vi "Send Set Power Setpoints.vi"(7 "Message Priority (Normal)":T1=enum."Normal", 8 "error in (no error)":errorcluster, 9 "Right Power Setpoint":dbl(slide) min=-1.0 max=1.0 step=0.1 scale=-1.0..1.0, 10 "Left Power Setpoint":dbl(slide) min=-1.0 max=1.0 step=0.1 scale=-1.0..1.0, 11 "Message Enqueuer":refnum<class "Message Enqueuer.lvclass">) -> (0 "error out":errorcluster, 3 "Message Enqueuer out":refnum<class "Message Enqueuer.lvclass">)   [LabVIEW 2014, in "Logical Systems.lvlib" / "Drive Train.lvlib" / "Set Power Setpoints Msg.lvclass"]
doc: "This VI sends the message to an actor."
uses:
  Set Power Setpoints Msg.lvclass
  <vilib>/ActorFramework/Message Enqueuer/Message Enqueuer.lvclass
  <vilib>/ActorFramework/Message Enqueuer/Message Priority.ctl
  Set Power Setpoints Msg.lvclass/Set Power Setpoints Msg.ctl
  <vilib>/ActorFramework/Message Enqueuer/Message Enqueuer.lvclass/Message Enqueuer.ctl
  <vilib>/ActorFramework/Message Priority Queue/Priority Enqueue.vi
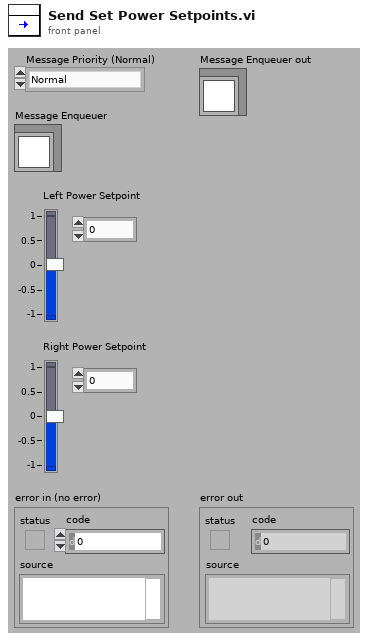
[diagram p1: front panel]
types:
  T1 = typedef "Actor Framework.lvlib/Message Enqueuer.lvclass/Message Priority.ctl" = enum16{"Low", "Normal", "High"}
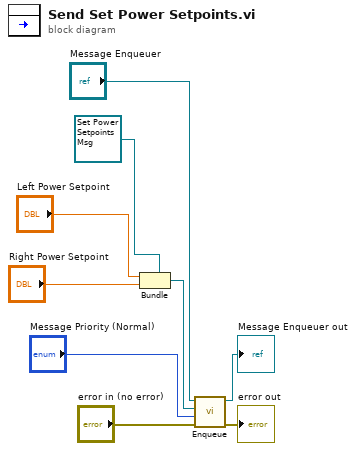
[diagram p0: block diagram]
diagram:
  n1 = Bundle(cluster=refnum<class "Set Power Setpoints Msg.lvclass"> refnum ("Object"), "Left Power Setpoint", "Right Power Setpoint") -> (w5:refnum<class "Set Power Setpoints Msg.lvclass">)
  n2 = call <vilib>:"Enqueue.vi"("error in (no error)"="error in (no error)", "Message Priority (Normal)"="Message Priority (Normal)", "Message"=w5, "Message Enqueuer in"="Message Enqueuer") -> ("error out"=→"error out":errorcluster, "Message Enqueuer out"=→"Message Enqueuer out":refnum<class "Message Enqueuer.lvclass">)  [unwired: 6 in]
